vi "main_init.vi"(0 "vi path":path, 11 "error in (no error)":errorcluster) -> (4 "Error log":refnum<vi>, 6 "Data acquisition":refnum<vi>, 15 "error out":errorcluster)   [LabVIEW 2023]
doc: "Initialize the basic startup VIs."
uses:
  task_1.lvlib
  Controls/event_operations.ctl
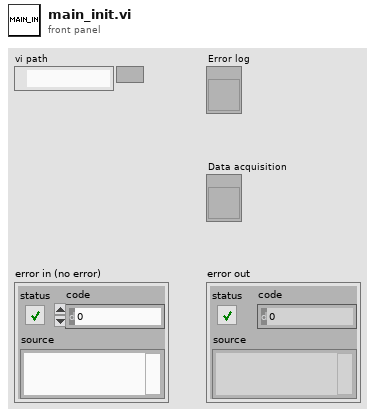
[diagram p1: front panel]
types:
  T1 = typedef "task_1.lvlib/event_operations.ctl" = enum16{"Create", "Generate", "Get_ref", "Destroy"}
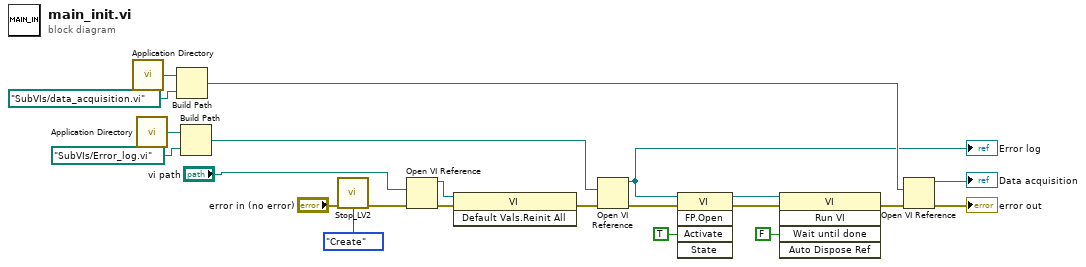
[diagram p0: block diagram]
diagram:
  n1 = call <vilib>:"Application Directory.vi"() -> ("Application Directory"=w22:path)
  n2 = call <vilib>:"Application Directory.vi"() -> ("Application Directory"=w14:path)
  n3 = Build Path(base path=w22, name or relative path=path "SubVIs/data_acquisition.vi") -> (appended path=w20:path)
  n4 = Build Path(base path=w14, name or relative path=path "SubVIs/Error_log.vi") -> (appended path=w13:path)
  n5 = call "Stop_LV2.vi"("error in (no error)"="error in (no error)", "Operations"=event_operations."Create") -> ("error out"=w3:errorcluster)  [unwired: 12 in, 1 out]
  n6 = Open VI Reference(vi path="vi path", error in (no error)=w3) -> (vi reference=w17:refnum<vi>, error out=w19:errorcluster)  [unwired: 4 in]
  n7 = invoke class="VI" method="Default Vals.Reinit All"(reference=w17, error in=w19) -> (error out=w18:errorcluster)  [unwired: 1 in, 2 out]
  n8 = Open VI Reference(vi path=w13, error in (no error)=w18) -> (vi reference=w7:refnum<vi>, error out=w16:errorcluster)  [unwired: 4 in]
  "Error log" <- w7
  n9 = invoke class="VI" method="FP.Open"(reference=w7, error in=w16, "Activate"=TRUE ("Activate?")) -> (reference out=w10:refnum<vi>, error out=w11:errorcluster)  [unwired: 2 in, 3 out]
  n10 = invoke class="VI" method="Run VI"(reference=w10, error in=w11, "Wait until done"=FALSE ("Wait Until Done")) -> (error out=w12:errorcluster)  [unwired: 2 in, 4 out]
  n11 = Open VI Reference(vi path=w20, error in (no error)=w12) -> (vi reference=→"Data acquisition":refnum<vi>, error out=→"error out":errorcluster)  [unwired: 4 in]
